vi "DAQ6363_PulseGenAcqV2.vi"(0 "APD2GTaskIn":refnum<k21>, 1 "APD1GTaskIn":refnum<k21>, 2 "APD1_On(T)":bool=TRUE, 3 "APD2_On(F)":bool, 4 "A2CntTaskIn":refnum<k21>, 5 "error in (no error)":errorcluster caption="entrée d'erreur (pas d'erreur)", 6 "A1CntTaskIn":refnum<k21>, 7 "HaltRef":refnum<vi>, 9 "SendTrig(T)":bool=TRUE, 10 "DataBindCtrlNm":string[](array[string]), 11 "Control Ref":refnum<vi>[](array[refnum])) -> (12 "A1CntTaskOut":refnum<k21>, 13 "A1Counts Out":u32 caption="A1CountsOut", 14 "APD2GTaskOut":refnum<k21>, 15 "APD1GTaskOut":refnum<k21>, 17 "A2Counts Out":u32 caption="A2CountsOut", 18 "A2CntTaskOut":refnum<k21>, 19 "error out":errorcluster caption="sortie d'erreur")   [LabVIEW 2019]
uses:
  <vilib>/DAQmx/read.llb/DAQmx Read (Counter U32 1Chan 1Samp).vi
  <vilib>/DAQmx/miscellaneous.llb/DAQmx Fill In Error Info.vi
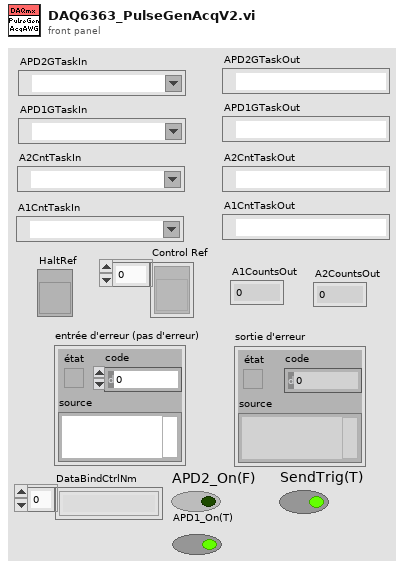
[diagram p1: front panel]
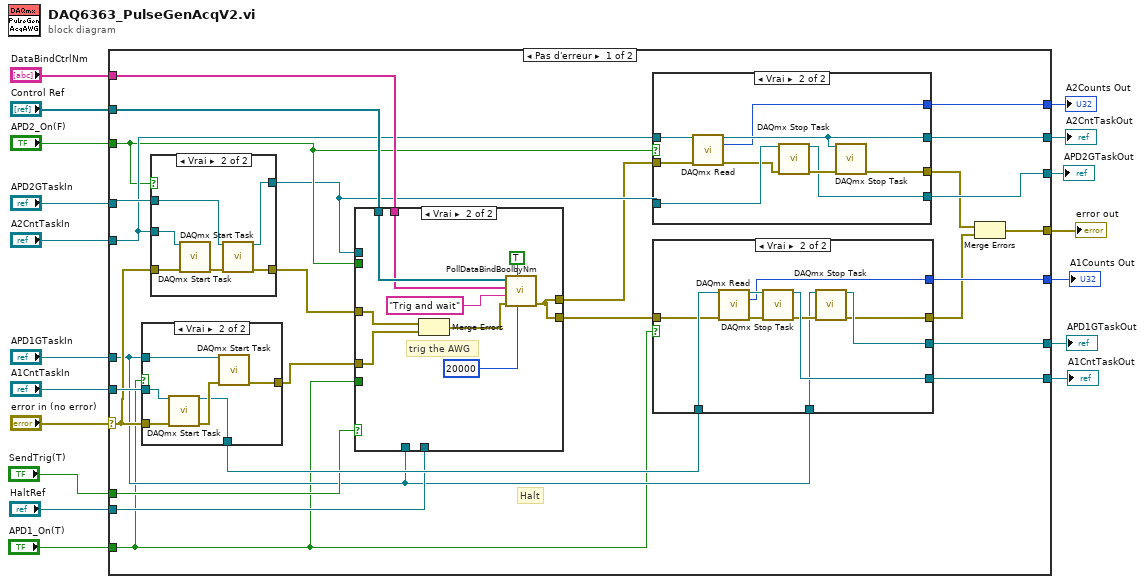
[diagram p0: block diagram]
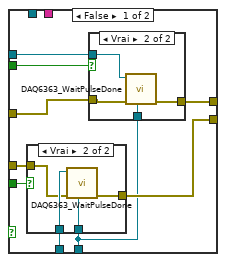
[diagram p4: hidden frame]
diagram:
  n1 = case shown="Pas d'erreur" "error in (no error)" {
    selector: "error in (no error)" -> [w26 w114]
    tunnel: [w21 w114] -> w16
    tunnel: "APD2GTaskIn" -> [w41 w118]
    tunnel: "A1CntTaskIn" -> [w42 w115]
    tunnel: "HaltRef" -> [w29 _]
    tunnel: "A2CntTaskIn" -> [w35 w116]
    tunnel: "APD1GTaskIn" -> [w23 w117]
    tunnel: [w40 _] -> w11
    tunnel: [w39 w118] -> w10
    tunnel: [w38 w115] -> w9
    tunnel: [w24 w117] -> w8
    tunnel: [w34 w116] -> w7
    tunnel: "Control Ref" -> [w37 _]
    tunnel: "DataBindCtrlNm" -> [w36 _]
    tunnel: [w33 _] -> w4
    tunnel: "APD2_On(F)" -> [w30 _]
    tunnel: "SendTrig(T)" -> [w31 _]
    tunnel: "APD1_On(T)" -> [w22 _]
    frame No Error {
      # "Halt"
      n2 = case shown="Vrai" w22 {
        tunnel: [w58 w65] -> w19
        tunnel: [w59 w63] -> w43
        tunnel: w42 -> [_ w62]
        tunnel: w26 -> [w58 w61]
        tunnel: w23 -> [w59 w60]
        frame False {
        }
        frame True {
          n3 = call <vilib>:"DAQmx Start Task.vi"("task/channels in"=w62, "error in"=w61) -> ("task out"=w63:refnum<k21>, "error out"=w64:errorcluster)  [unwired: 12 in]
          n4 = call <vilib>:"DAQmx Start Task.vi"("task/channels in"=w60, "error in"=w64) -> ("error out"=w65:errorcluster)  [unwired: 12 in, 1 out]
        }
      }
      n5 = case shown="Vrai" w30 {
        tunnel: w26 -> [w106 w112]
        tunnel: [w106 w111] -> w44
        tunnel: w41 -> [w107 w110]
        tunnel: w35 -> [_ w109]
        tunnel: [w107 w108] -> w27
        frame False {
        }
        frame True {
          n6 = call <vilib>:"DAQmx Start Task.vi"("task/channels in"=w109, "error in"=w112) -> ("error out"=w113:errorcluster)  [unwired: 12 in, 1 out]
          n7 = call <vilib>:"DAQmx Start Task.vi"("task/channels in"=w110, "error in"=w113) -> ("task out"=w108:refnum<k21>, "error out"=w111:errorcluster)  [unwired: 12 in]
        }
      }
      n8 = case shown="Vrai" w31 {
        tunnel: w44 -> [w72 w93]
        tunnel: w37 -> [_ w89]
        tunnel: w36 -> [_ w88]
        tunnel: [w69 w87] -> w32
        tunnel: w30 -> [w73 _]
        tunnel: w23 -> [w74 _]
        tunnel: w29 -> [w68 _]
        tunnel: w27 -> [w71 _]
        tunnel: [w70 w87] -> w25
        tunnel: w22 -> [w67 _]
        tunnel: w19 -> [w66 w85]
        frame False {
          n9 = case shown="Vrai" w67 {
            tunnel: w74 -> [_ w79]
            tunnel: w68 -> [_ w78]
            tunnel: [w75 w77] -> w69
            tunnel: w66 -> [w75 w76]
            frame False {
            }
            frame True {
              n10 = call <userlib>:"DAQ6363_WaitPulseDone.vi"("HaltRef"=w78, "error in (no error)"=w76, "TaskIn"=w79) -> ("error out"=w77:errorcluster)  [unwired: 7 in, 1 out]
            }
          }
          n11 = case shown="Vrai" w73 {
            tunnel: w72 -> [w80 w84]
            tunnel: [w80 w83] -> w70
            tunnel: w71 -> [_ w82]
            tunnel: w68 -> [_ w81]
            frame False {
            }
            frame True {
              n12 = call <userlib>:"DAQ6363_WaitPulseDone.vi"("HaltRef"=w81, "error in (no error)"=w84, "TaskIn"=w82) -> ("error out"=w83:errorcluster)  [unwired: 7 in, 1 out]
            }
          }
        }
        frame True {
          # "trig the AWG"
          n13 = Merge Errors(w93, w85) -> (w86:errorcluster)
          n14 = call <userlib>:"PollDataBindBoolbyNm.vi"("Timeout(ms)"=20000, "Valeur"=TRUE, "error in"=w86, "TargetName"="Trig and wait", "DataBindCtrlNm"=w88, "Control Ref"=w89) -> ("error out"=w87:errorcluster)  [unwired: 4 in, 1 out]
        }
      }
      n15 = case shown="Vrai" w30 {
        tunnel: [w94 w104] -> w39
        tunnel: w35 -> [w95 w103]
        tunnel: [w95 w102] -> w34
        tunnel: w27 -> [w94 w101]
        tunnel: [_ w100] -> w33
        tunnel: [w96 w99] -> w28
        tunnel: w25 -> [w96 w97]
        frame False {
        }
        frame True {
          n16 = call-poly <vilib>:"DAQmx Read.vi"("task/channels in"=w103, "error in"=w97) -> ("task out"=w102:refnum<k21>, "data"=w100:u32, "error out"=w98:errorcluster)  [unwired: 11 in]
          n17 = call <vilib>:"DAQmx Stop Task.vi"("task/channels in"=w101, "error in"=w98) -> ("task out"=w104:refnum<k21>, "error out"=w105:errorcluster)  [unwired: 12 in]
          n18 = call <vilib>:"DAQmx Stop Task.vi"("task/channels in"=w102, "error in"=w105) -> ("error out"=w99:errorcluster)  [unwired: 12 in, 1 out]
        }
      }
      n19 = case shown="Vrai" w22 {
        tunnel: w43 -> [w46 w57]
        tunnel: [_ w54] -> w40
        tunnel: [w46 w53] -> w38
        tunnel: w32 -> [w45 w51]
        tunnel: w23 -> [w47 w50]
        tunnel: [w47 w49] -> w24
        tunnel: [w45 w48] -> w20
        frame False {
        }
        frame True {
          n20 = call-poly <vilib>:"DAQmx Read.vi"("task/channels in"=w57, "error in"=w51) -> ("task out"=w55:refnum<k21>, "data"=w54:u32, "error out"=w56:errorcluster)  [unwired: 11 in]
          n21 = call <vilib>:"DAQmx Stop Task.vi"("task/channels in"=w55, "error in"=w56) -> ("task out"=w53:refnum<k21>, "error out"=w52:errorcluster)  [unwired: 12 in]
          n22 = call <vilib>:"DAQmx Stop Task.vi"("task/channels in"=w50, "error in"=w52) -> ("task out"=w49:refnum<k21>, "error out"=w48:errorcluster)  [unwired: 12 in]
        }
      }
      n23 = Merge Errors(w28, w20) -> (w21:errorcluster)
    }
    frame Error {
    }
  }
  "error out" <- w16
  "APD2GTaskOut" <- w10
  "A1Counts Out" <- w11
  "A2CntTaskOut" <- w7
  "A1CntTaskOut" <- w9
  "APD1GTaskOut" <- w8
  "A2Counts Out" <- w4
